vi "DeploymentTest-ModifiedTiming.vi"() -> ()   [LabVIEW 2018]
uses:
  <vilib>/myRIO/Instrument Drivers/Onboard IO/DIO/typedefs/DIO Reference.ctl
  <vilib>/myRIO/Common/Instrument Driver Framework/Utilities/typedefs/myRIO Generic Hardware Reference.ctl
  <vilib>/myRIO/Common/Instrument Driver Framework/Utilities/typedefs/Hardware Version Enum.ctl
  <vilib>/myRIO/Common/Instrument Driver Framework/Utilities/typedefs/myRIO v1.0 Reference.ctl
  <vilib>/myRIO/Common/Instrument Driver Framework/Utilities/typedefs/Generic FPGA Reference.ctl
  <vilib>/myRIO/Common/Instrument Driver Framework/myRIO v1.0/DIO/typedefs/DIO Channels List.ctl
  <vilib>/myRIO/Common/Instrument Driver Framework/myRIO v1.0/DIO/typedefs/DIO Channels Enum.ctl
  <vilib>/userdefined/High Color/nirio_resource_hc.ctl
  <vilib>/myRIO/Common/Instrument Driver Framework/Utilities/vis/Is FPGA Ref Available.vi
  <vilib>/myRIO/Common/Instrument Driver Framework/myRIO v1.0/DIO/vis/myRIO v1.1 Open DIO.vi
  <vilib>/myRIO/Instrument Drivers/Onboard IO/DIO/vis/Read.vi
  <vilib>/myRIO/Instrument Drivers/Onboard IO/DIO/vis/Write.vi
  <vilib>/myRIO/Common/Instrument Driver Framework/Utilities/vis/Validate Channels.vi
  <vilib>/myRIO/Common/Instrument Driver Framework/myRIO v1.0/DIO/vis/myRIO v1.0 Reserve DIO.vi
  <vilib>/myRIO/Common/Instrument Driver Framework/myRIO v1.0/UART/vis/myRIO v1.0 Close UART.vi
  <vilib>/myRIO/Common/Instrument Driver Framework/myRIO v1.0/Resource Manager/vis/myRIO v1.0 Reserve Channel List.vi
  <vilib>/myRIO/Common/Instrument Driver Framework/myRIO v1.0/DIO/vis/myRIO v1.0 Build MUX Configuration DIO.vi
  <vilib>/myRIO/Common/Instrument Driver Framework/myRIO v1.0/Resource Manager/vis/myRIO v1.0 Reserve Channel.vi
  <vilib>/myRIO/Common/Instrument Driver Framework/myRIO v1.0/Resource Manager/vis/myRIO v1.0 Unreserve Channel.vi
  <vilib>/myRIO/Common/Instrument Driver Framework/myRIO v1.0/Resource Manager/vis/myRIO v1.0 Create Configuration List.vi
  <vilib>/myRIO/Common/Instrument Driver Framework/myRIO v1.0/Resource Manager/vis/myRIO v1.0 Build Mutex Name.vi
  <vilib>/Utility/VariantDataType/GetNumericInfo.vi
  <vilib>/Utility/error.llb/Error Cluster From Error Code.vi
  <vilib>/myRIO/Common/Instrument Driver Framework/myRIO v1.0/myRIO v1.1 Open.vi
  <vilib>/myRIO/Common/Instrument Driver Framework/Utilities/vis/IO Manager.vi
  <vilib>/myRIO/Common/Instrument Driver Framework/Utilities/vis/Configuration Manager.vi
  <vilib>/myRIO/Common/Instrument Driver Framework/myRIO v1.0/Resource Manager/vis/myRIO v1.0 Configure IO.vi
  <vilib>/myRIO/Common/Instrument Driver Framework/myRIO v1.0/myRIO v1.0 Close.vi
  <vilib>/myRIO/Common/Instrument Driver Framework/myRIO v1.0/DIO/vis/myRIO v1.0 Read DIO.vi
  <vilib>/functionblocks/Edge Detection/Edge Detect/Edge Detect.vi
  <vilib>/myRIO/Common/Instrument Driver Framework/myRIO v1.0/DIO/vis/myRIO v1.0 Write DIO.vi
  <vilib>/functionblocks/Edge Detection/One Shot Rising with Input/One Shot Rising with Input.vi
  <vilib>/myRIO/Common/Instrument Driver Framework/Utilities/vis/FPGA Ref Manager.vi
  <vilib>/myRIO/Common/Instrument Driver Framework/myRIO v1.0/myRIO v1.0 Reset FPGA.vi
  <vilib>/myRIO/Common/Instrument Driver Framework/myRIO v1.0/IRQ/vis/myRIO v1.0 IRQ Info FGV.vi
  <vilib>/myRIO/Common/Instrument Driver Framework/myRIO v1.0/IRQ/vis/myRIO v1.0 Timer IRQ Info FGV.vi
  <vilib>/myRIO/Common/Instrument Driver Framework/myRIO v1.0/IRQ/vis/myRIO v1.0 ISR Agent.vi
  <vilib>/myRIO/Express VI/Onboard IO/DI/DI Express VI.xnode
  <vilib>/myRIO/Instrument Drivers/Onboard IO/DIO/vis/myRIO DIO Open.xnode
  <vilib>/functionblocks/FB Core/FB Core.xnode
  <vilib>/myRIO/Express VI/Onboard Devices/LED/LED Express VI.xnode
  <vilib>/myRIO/Express VI/Onboard Devices/Button/Button Express VI.xnode
  <vilib>/myRIO/Express VI/Onboard IO/DO/DO Express VI.xnode
  <vilib>/myRIO/Instrument Drivers/Onboard IO/DIO/DIO.lvlib
  <vilib>/functionblocks/NI_FunctionBlock Libraries.lvlib
  <vilib>/myRIO/Instrument Drivers/Utilities/Utilities.lvlib
panel:
  out "HalfRevT":dbl
  out "Elapsed Time (s)":dbl
  out "In correct Half":bool
  out "Solenoid Engaged":bool
  out "DeltaT":dbl=0.25
  out "Wait Time":dbl format="%.2f"
  out "InYBKHalf":bool=TRUE
  out "Yellow-Black Half?":bool
  out "T Known":bool=TRUE
  out "Clicks":i32
  out "nanners":bool
  out "Current Height":string
  out "Color":string
  out "Our Team Num":i32
  out "Yellow":bool
  out "Blue":bool
  out "Total Time":dbl caption="Elapsed Time (s)"
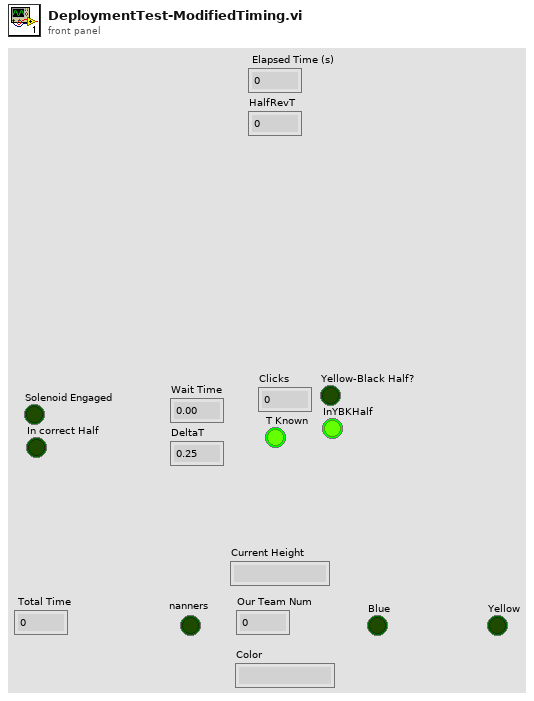
[diagram p1: front panel]
types:
  T1 = typedef "DIO.lvlib/DIO Reference.ctl" = cluster{"myRIO Reference":T2, "DIO Channels List":T6}
  T2 = typedef "myRIO Generic Hardware Reference.ctl" = cluster{"myRIO Model":T3, "myRIO Hardware Reference":T4}
  T3 = typedef "Hardware Version Enum.ctl" = enum16{"Unknown", "myRIO-1900", "myRIO-1950", "roboRIO", "NI ELVIS RIO CM", "ELVIS III"}
  T4 = typedef "myRIO v1.0 Reference.ctl" = cluster{"Generic FPGA Reference":T5, "Allow multiple opens":bool}
  T5 = typedef "Generic FPGA Reference.ctl" = refnum<k20>
  T6 = typedef "DIO Channels List.ctl" = T7[]
  T7 = typedef "DIO Channels Enum.ctl" = enum16{"Not Connected", "C/DIO0", "C/DIO1", "C/DIO2", "C/DIO3", "C/DIO4", "C/DIO5", "C/DIO6", "C/DIO7", "A/DIO0", "A/DIO1", "A/DIO2", "A/DIO3", "A/DIO4", "A/DIO5", "A/DIO6", "A/DIO7", "A/DIO8", "A/DIO9", "A/DIO10", "A/DIO11", "A/DIO12", "A/DIO13", "A/DIO14", "A/DIO15", "A/DIO16", "A/DIO17", "A/DIO18", "A/DIO19", "B/DIO0", "B/DIO1", "B/DIO2", "B/DIO3", "B/DIO4", "B/DIO5", "B/DIO6", "B/DIO7", "B/DIO8", "B/DIO9", "B/DIO10", "B/DIO11", "B/DIO12", "B/DIO13", "B/DIO14", "B/DIO15", "B/DIO16", "B/DIO17", "B/DIO18", "B/DIO19", "LED0", "LED1", "LED2", "LED3", "Button0", "DIO/DIO0", "DIO/DIO1", "DIO/DIO2", "DIO/DIO3", "DIO/DIO4", "DIO/DIO5", "DIO/DIO6", "DIO/DIO7", "DIO/DIO8", "DIO/DIO9", "SPI/CS0", "SPI/CS1", "SPI/CS2", "SPI/CS3", "LED RADIO (Green)", "LED RADIO (Red)", "LED COMM (Green)", "LED COMM (Red)", "LED MODE (Green)", "LED MODE (Red)"}
  T8 = typedef "nirio_resource_hc.ctl" = tag
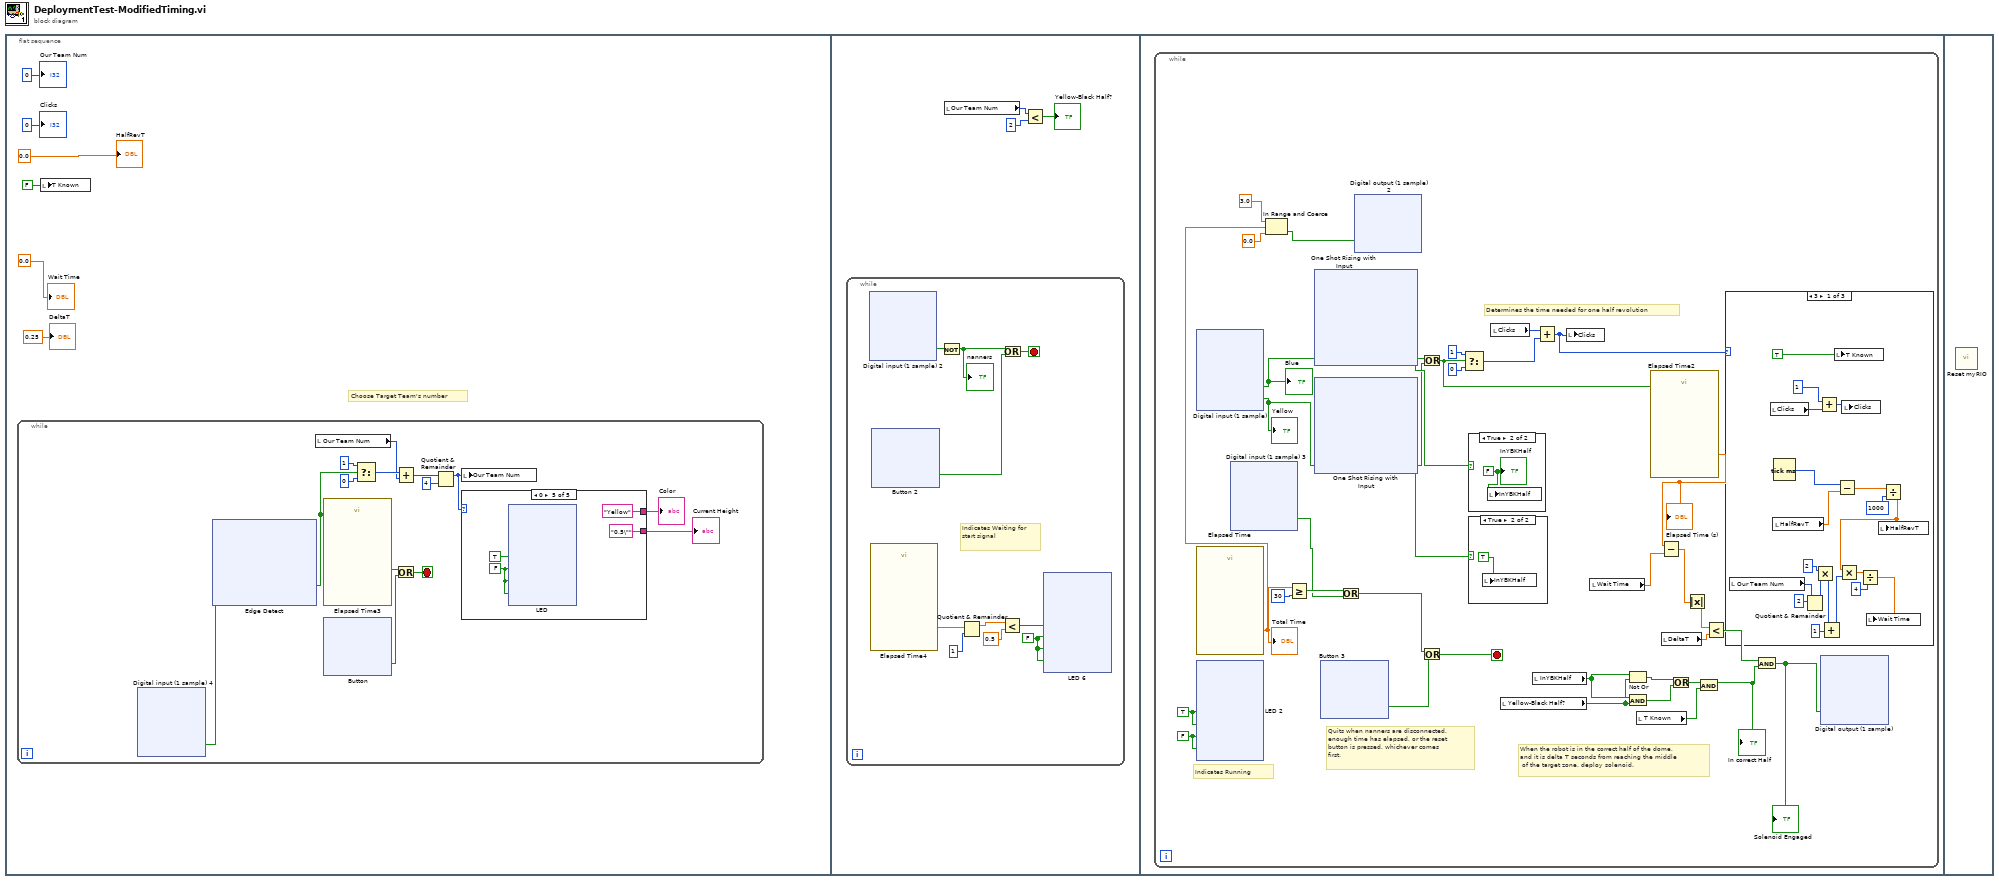
[diagram p0: block diagram]
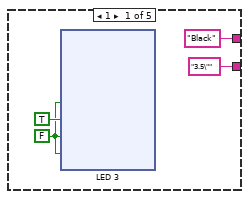
[diagram p2: hidden frame]
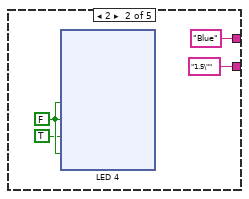
[diagram p3: hidden frame]
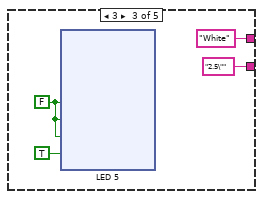
[diagram p4: hidden frame]
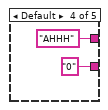
[diagram p5: hidden frame]
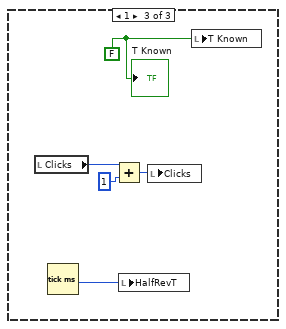
[diagram p9: hidden frame]
diagram:
  n1 = flat-sequence {
    frame #0 {
      # "Choose Target Team's number"
      n2 = while {
        stop <- w10 stop-if-true
        n3 = xnode "Digital input (1 sample) 4"() -> ("Big Red Button (B/DIO1 (Pin 13))"=w8:bool)  [unwired: 1 in, 1 out]
        n4 = xnode "Edge Detect"("input 2"=w8, "input 1"=w8) -> ("output"=w7:bool)  [unwired: 1 in, 1 out]
        n5 = local read "Our Team Num"() -> (w15:i32)
        n6 = call "Elapsed Time3"("Reset"=w7) -> ("Time has Elapsed"=w13:bool)  [unwired: 11 in, 7 out]
        n7 = xnode "Button"() -> ("Value"=w9:bool)  [unwired: 1 in, 1 out]
        n8 = Select(t=1, s=w7, f=0) -> (s? t:f=w18:i32)
        n9 = Add(x=w18, y=w15) -> (x+y=w17:i32)
        n10 = Or(x=w13, y=w9) -> (x .or. y?=w10:bool)
        n11 = Quotient & Remainder(x=w17, y=4) -> (x-y*floor(x/y)=w14:i32)  [unwired: 1 out]
        n12 = local write "Our Team Num"(w14) -> ()
        n13 = case shown="0" w14 {
          tunnel: ["Black" "Blue" "White" "AHHH" "Yellow"] -> w12
          tunnel: ["3.5\"" "1.5\"" "2.5\"" "0" "0.5\""] -> w11
          frame 1 {
            w57 = FALSE
            n14 = xnode "LED 3"("LED0"=w57, "LED1"=TRUE, "LED2"=w57, "LED3"=w57) -> ()  [unwired: 1 in, 1 out]
          }
          frame 2 {
            w101 = FALSE
            n15 = xnode "LED 4"("LED0"=w101, "LED1"=w101, "LED2"=TRUE, "LED3"=w101) -> ()  [unwired: 1 in, 1 out]
          }
          frame 3 {
            w142 = FALSE
            n16 = xnode "LED 5"("LED0"=w142, "LED1"=w142, "LED2"=w142, "LED3"=TRUE) -> ()  [unwired: 1 in, 1 out]
          }
          frame Default {
          }
          frame 0 {
            w186 = FALSE
            n17 = xnode "LED"("LED0"=TRUE, "LED1"=w186, "LED2"=w186, "LED3"=w186) -> ()  [unwired: 1 in, 1 out]
          }
        }
        "Color" <- w12
        "Current Height" <- w11
      }
      n18 = local write "T Known"(FALSE) -> ()
      "Our Team Num" <- 0
      "Clicks" <- 0
      "Wait Time" <- 0.0
      "DeltaT" <- 0.25
      "HalfRevT" <- 0.0
    }
    frame #1 {
      n19 = while {
        stop <- w313 stop-if-true
        w309 = FALSE
        # "Indicates Waiting for start signal"
        n20 = xnode "Digital input (1 sample) 2"() -> ("B/DIO0 (Pin 11)"=w315:bool)  [unwired: 1 in, 1 out]
        n21 = call "Elapsed Time4"() -> ("Elapsed Time (s)"=w311:dbl)  [unwired: 12 in, 7 out]
        n22 = xnode "Button 2"() -> ("Value"=w312:bool)  [unwired: 1 in, 1 out]
        n23 = Not(x=w315) -> (.not. x?=w314:bool)
        "nanners" <- w314
        n24 = Quotient & Remainder(x=w311, y=1) -> (x-y*floor(x/y)=w308:dbl)  [unwired: 1 out]
        n25 = Less?(x=w308, y=0.5) -> (x < y?=w306:bool)
        n26 = Or(x=w314, y=w312) -> (x .or. y?=w313:bool)
        n27 = xnode "LED 6"("LED0"=w306, "LED1"=w309, "LED2"=w309, "LED3"=w309) -> ()  [unwired: 1 in, 1 out]
      }
      n28 = local read "Our Team Num"() -> (w304:i32)
      n29 = Less?(x=w304, y=2) -> (x < y?=→"Yellow-Black Half?":bool)
    }
    frame #2 {
      n30 = while {
        stop <- w426 stop-if-true
        w455 = FALSE
        w456 = TRUE
        # "Quits when nanners are disconnected, \nenough time has elapsed, or the reset\nbutton is pressed, whichever comes \nfirst."
        # "When the robot is in the correct half of the dome, \nand it is delta T seconds from reaching the middle\n of the target zone, deploy solenoid."
        # "Determines the time needed for one half revolution"
        # "Indicates Running"
        n31 = xnode "Digital input (1 sample)"() -> ("Blue (DI1) (B/DIO5 (Pin 21))"=w449:bool, "Yellow (DI2) (B/DIO2 (Pin 15))"=w424:bool)  [unwired: 1 in, 1 out]
        "Blue" <- w449
        "Yellow" <- w424
        n32 = call "Elapsed Time"() -> ("Elapsed Time (s)"=w428:dbl)  [unwired: 12 in, 7 out]
        "Total Time" <- w428
        n33 = xnode "LED 2"("LED0"=w456, "LED1"=w456, "LED2"=w455, "LED3"=w455) -> ()  [unwired: 1 in, 1 out]
        n34 = xnode "Digital input (1 sample) 3"() -> ("Nanners (B/DIO0 (Pin 11))"=w425:bool)  [unwired: 1 in, 1 out]
        n35 = In Range and Coerce(upper limit=3.0, x=w428, lower limit=0.0) -> (In Range?=w429:bool)  [unwired: 1 out]
        n36 = Greater Or Equal?(x=w428, y=30) -> (x >= y?=w458:bool)
        n37 = xnode "One Shot Rising with Input"("input"=w449) -> ("output"=w448:bool)  [unwired: 1 in, 1 out]
        n38 = xnode "One Shot Rising with Input"("input"=w424) -> ("output"=w447:bool)  [unwired: 1 in, 1 out]
        n39 = xnode "Button 3"() -> ("Value"=w450:bool)  [unwired: 1 in, 1 out]
        n40 = Or(x=w458, y=w425) -> (x .or. y?=w457:bool)
        n41 = xnode "Digital output (1 sample) 2"("A/DIO2 (Pin 15)"=w429) -> ()  [unwired: 1 in, 1 out]
        n42 = Or(x=w448, y=w447) -> (x .or. y?=w432:bool)
        n43 = Or(x=w457, y=w450) -> (x .or. y?=w426:bool)
        n44 = Select(t=1, s=w432, f=0) -> (s? t:f=w451:i32)
        n45 = case shown="True" w447 {
          frame False {
          }
          frame True {
            n46 = local write "InYBKHalf"(TRUE) -> ()
          }
        }
        n47 = case shown="True" w448 {
          frame False {
          }
          frame True {
            w531 = FALSE
            n48 = local write "InYBKHalf"(w531) -> ()
            "InYBKHalf" <- w531
          }
        }
        n49 = local read "Clicks"() -> (w454:i32)
        n50 = local read "Yellow-Black Half?"() -> (w445:bool)
        n51 = local read "InYBKHalf"() -> (w446:bool)
        n52 = Add(x=w454, y=w451) -> (x+y=w433:i32)
        n53 = local write "Clicks"(w433) -> ()
        n54 = local read "Wait Time"() -> (w442:dbl)
        n55 = Not Or(1:w445, 2:w446) -> (0:w444:bool)
        n56 = And(x=w446, y=w445) -> (x .and. y?=w443:bool)
        n57 = local read "T Known"() -> (w434:bool)
        n58 = call "Elapsed Time2"("Reset"=w432) -> ("Elapsed Time (s)"=w436:dbl)  [unwired: 11 in, 7 out]
        "Elapsed Time (s)" <- w436
        n59 = Subtract(x=w436, y=w442) -> (x-y=w441:dbl)
        n60 = local read "DeltaT"() -> (w439:dbl)
        n61 = Or(x=w444, y=w443) -> (x .or. y?=w437:bool)
        n62 = Absolute Value(x=w441) -> (abs(x)=w440:dbl)
        n63 = And(x=w437, y=w434) -> (x .and. y?=w435:bool)
        "In correct Half" <- w435
        n64 = Less?(x=w440, y=w439) -> (x < y?=w438:bool)
        n65 = case shown="3" w433 {
          frame 3 {
            n66 = local read "Our Team Num"() -> (w582:i32)
            n67 = local read "Clicks"() -> (w575:i32)
            n68 = local read "HalfRevT"() -> (w584:dbl)
            n69 = Tick Count (ms)() -> (millisecond timer value=w583:u32)
            n70 = Quotient & Remainder(x=w582, y=2) -> (x-y*floor(x/y)=w580:i32)  [unwired: 1 out]
            n71 = Multiply(x=2, y=w580) -> (x*y=w572:i32)
            n72 = Add(x=1, y=w575) -> (x+y=w573:i32)
            n73 = Add(x=w572, y=1) -> (x+y=w570:i32)
            n74 = local write "T Known"(TRUE) -> ()
            n75 = Subtract(x=w583, y=w584) -> (x-y=w576:dbl)
            n76 = local write "Clicks"(w573) -> ()
            n77 = Divide(x=w576, y=1000) -> (x/y=w567:dbl)
            n78 = Multiply(x=w567, y=w570) -> (x*y=w579:dbl)
            n79 = Divide(x=w579, y=4) -> (x/y=w577:dbl)
            n80 = local write "Wait Time"(w577) -> ()
            n81 = local write "HalfRevT"(w567) -> ()
          }
          frame Default {
          }
          frame 1 {
            w590 = FALSE
            n82 = local read "Clicks"() -> (w588:i32)
            n83 = Tick Count (ms)() -> (millisecond timer value=w589:u32)
            n84 = Add(x=w588, y=1) -> (x+y=w586:i32)
            n85 = local write "HalfRevT"(w589) -> ()
            n86 = local write "Clicks"(w586) -> ()
            n87 = local write "T Known"(w590) -> ()
            "T Known" <- w590
          }
        }
        n88 = And(x=w438, y=w435) -> (x .and. y?=w427:bool)
        "Solenoid Engaged" <- w427
        n89 = xnode "Digital output (1 sample)"("A/DIO1 (Pin 13)"=w427) -> ()  [unwired: 1 in, 1 out]
      }
    }
    frame #3 {
      n90 = call <vilib>:"Reset myRIO.vi"() -> ()  [unwired: 11 in, 1 out]
    }
  }
